vi "Screen_Cycle_state.vi"(11 "PLC to Labview Data":i32[](array[numeric])) -> (3 "Cyc St":bool[](array[boolean]))   [LabVIEW 2017]
uses:
  53695393-22c5-4a09-a575-66eec6b345ad.vi
  a48b5781-5004-46dc-a403-898a4e6365e6.vi
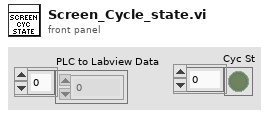
[diagram p1: front panel]
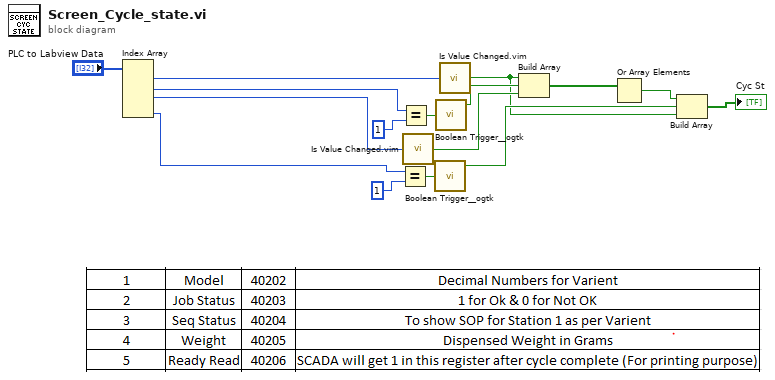
[diagram p0: block diagram]
diagram:
  n1 = Index Array(array="PLC to Labview Data") -> (element #1=w16:i32, element #2=w14:i32, element #3=w10:i32, element #5=w6:i32)  [unwired: 5 in, 1 out]
  n2 = Equal?(x=w6, y=1) -> (x = y?=w8:bool)
  n3 = Equal?(x=w14, y=1) -> (x = y?=w12:bool)
  n4 = call "Is Value Changed.vim"("value"=w10) -> ("changed or first call?"=w9:bool)
  n5 = call <userlib>:"Boolean Trigger__ogtk.vi"("Boolean Input"=w8) -> ("Rising Edge"=w4:bool)  [unwired: 1 in, 1 out]
  n6 = call <userlib>:"Boolean Trigger__ogtk.vi"("Boolean Input"=w12) -> ("Rising Edge"=w11:bool)  [unwired: 1 in, 1 out]
  n7 = call "Is Value Changed.vim"("value"=w16) -> ("changed or first call?"=w1:bool)
  n8 = Build Array(w1, w11, w9) -> (w5:bool[])
  n9 = Or Array Elements(Boolean array=w5) -> (logical OR=w3:bool)
  n10 = Build Array(w3, w4, w1) -> (→"Cyc St":bool[])
